vi "Maximum Power.vi"(9 "Current (Amps) vs Voltage (Volts)":cluster{"voltage":dbl[], "current":dbl[]}(graph)) -> (2 "max power":dbl, 3 "Power (Watts) vs Voltage (Volts)":cluster{"voltage":dbl[], dbl[]}(graph), 4 "current at max power":dbl, 6 "voltage at max power":dbl)   [LabVIEW 2016]
panel:
  out "current":dbl[](array[numeric])
  out "voltage":dbl[](array[numeric])
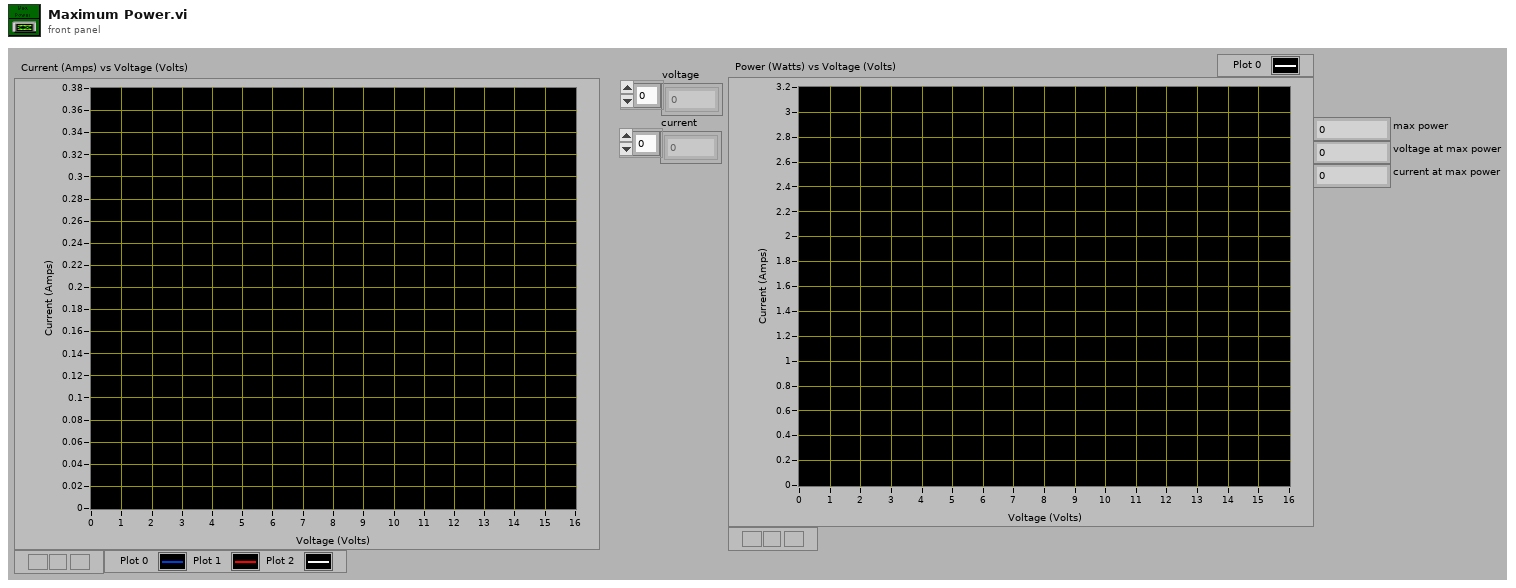
[diagram p1: front panel]
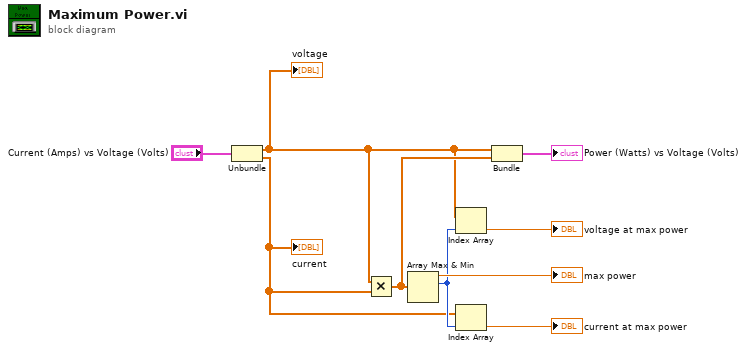
[diagram p0: block diagram]
diagram:
  n1 = Unbundle("Current (Amps) vs Voltage (Volts)") -> ("voltage"=w4:dbl[], "current"=w3:dbl[])
  "voltage" <- w4
  "current" <- w3
  n2 = Multiply(x=w4, y=w3) -> (x*y=w7:dbl[])
  n3 = Array Max & Min(array=w7) -> (max value=→"max power":dbl, max index (indices)=w8:i32)  [unwired: 2 out]
  n4 = Index Array(array=w4, index=w8) -> (element=→"voltage at max power":dbl)
  n5 = Index Array(array=w3, index=w8) -> (element=→"current at max power":dbl)
  n6 = Bundle("voltage"=w4, w7) -> (→"Power (Watts) vs Voltage (Volts)":cluster{"voltage":dbl[], dbl[]})  [unwired: 1 out]
